vi "setFPGAReference.vi"(10 "FPGAReference":refnum<k20>, 11 "MyHealthAndStatusWriteFIFO in":refnum<class "MyHealthAndStatusWriteFIFO.lvclass">) -> (3 "MyHealthAndStatusWriteFIFO out":refnum<class "MyHealthAndStatusWriteFIFO.lvclass">)   [LabVIEW 2015, in "MyHealthAndStatusWriteFIFO.lvclass"]
uses:
  MyHealthAndStatusWriteFIFO.lvclass
  MyHealthAndStatusWriteFIFO.lvclass/MyHealthAndStatusWriteFIFO.ctl
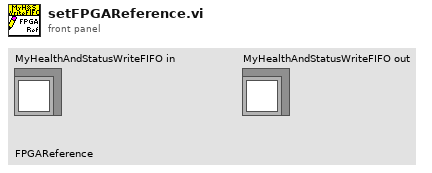
[diagram p1: front panel]
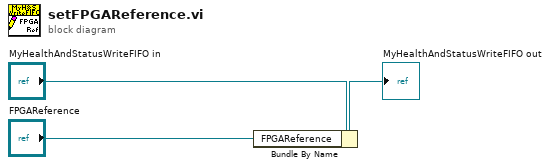
[diagram p0: block diagram]
diagram:
  n1 = Bundle By Name(cluster="MyHealthAndStatusWriteFIFO in", "FPGAReference"="FPGAReference") -> (→"MyHealthAndStatusWriteFIFO out":refnum<class "MyHealthAndStatusWriteFIFO.lvclass">)
